vi "AutoCAD busy.vi"(6 "error in (no error)":errorcluster, 7 "Application":refnum<k7>) -> (2 "error out":errorcluster, 3 "IsQuiescent":bool)   [LabVIEW 2015]
panel:
  out "Numeric":i32
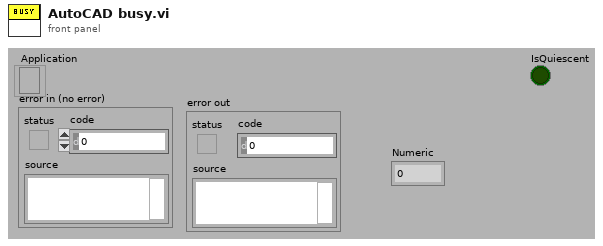
[diagram p1: front panel]
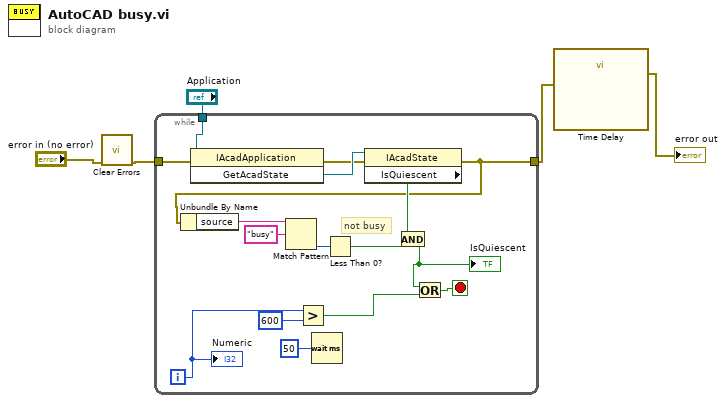
[diagram p0: block diagram]
diagram:
  n1 = call <vilib>:"Clear Errors.vi"("error in (no error)"="error in (no error)") -> ("error out"=w3:errorcluster)  [unwired: 5 in, 1 out]
  n2 = while {
    tunnel: "Application" -> [w21]
    tunnel: w3 -> [w12]
    tunnel: [w11] -> w2
    i -> [w15]
    stop <- w14 stop-if-true
    # "not busy"
    n3 = invoke class="IAcadApplication" method="GetAcadState"(reference=w21, error in=w12) -> (error out=w19:errorcluster, "GetAcadState"=w20:refnum<k7>)  [unwired: 1 in, 1 out]
    n4 = Greater?(x=w15, y=600) -> (0:w17:bool)
    n5 = Wait (ms)(milliseconds to wait=u32 50) -> ()  [unwired: 1 out]
    n6 = property class="IAcadState"(reference=w20, error in=w19) -> (error out=w11:errorcluster, "IsQuiescent"=w13:bool)  [unwired: 1 out]
    n7 = Unbundle By Name(w11) -> ("source"=w10:string)
    n8 = Match Pattern(string=w10, regular expression="busy") -> (offset past match=w8:i32)  [unwired: 1 in, 3 out]
    n9 = Less Than 0?(x=w8) -> (x < 0?=w7:bool)
    n10 = And(x=w13, y=w7) -> (x .and. y?=w6:bool)
    "IsQuiescent" <- w6
    n11 = Or(x=w6, y=w17) -> (x .or. y?=w14:bool)
    "Numeric" <- w15
  }
  n12 = call "Time Delay"("error in (no error)"=w2) -> ("error out"=→"error out":errorcluster)  [unwired: 10 in]
